vi "Sos_2024.vi"(0 "Temperature (K)":dbl=293.15 format="%.4g", 2 "Type of air":i32(listbox)=4, 5 "CO2 content (ppm)":dbl=500.0, 8 "Pressure (Pa)":dbl=101325.0 format="%.1f", 10 "xw molar fraction water vapor":dbl format="%.7g", 15 "Frequency (Hz)":dbl) -> (3 "virial correction Kv (ppm)":dbl=506.9979263453592, 6 "heat capacity correction Kc (ppm)":dbl=-1069.8067159622403 format="%.1f", 7 "relaxation correction Kr (ppm)":dbl=258.42726337360375 format="%#.0f", 12 "simple speed of sound":dbl=344.29226419685074 format="%.4f", 13 "heat & virial & relax corrected speed of sound humid air":dbl=344.2397436562656 format="%.4f", 14 "heat capacity corrected speed of sound [m/s]":dbl=344.10805182751363 format="%.4f", 17 "heat capacity & virial corrected speed of sound":dbl=344.19527180818477 format="%.4f")   [LabVIEW 2016]
panel:
  # "m/s"
  # "m/s"
  # "m/s"
  # "m/s"
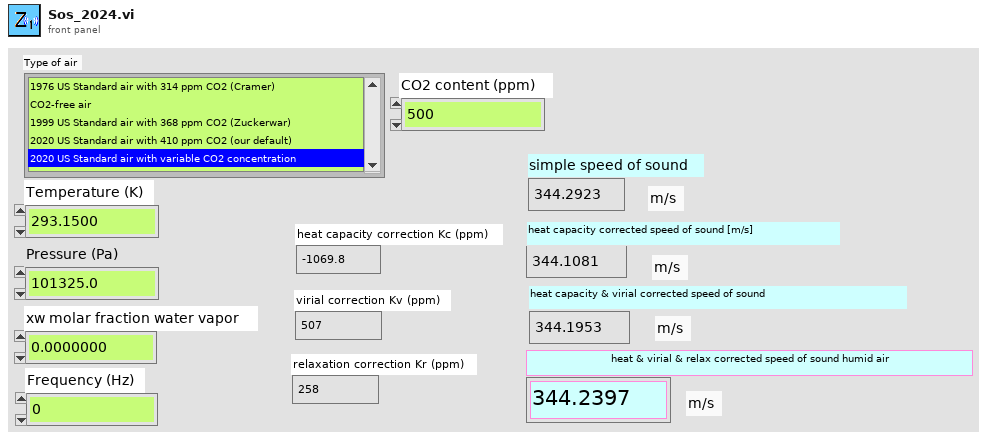
[diagram p1: front panel]
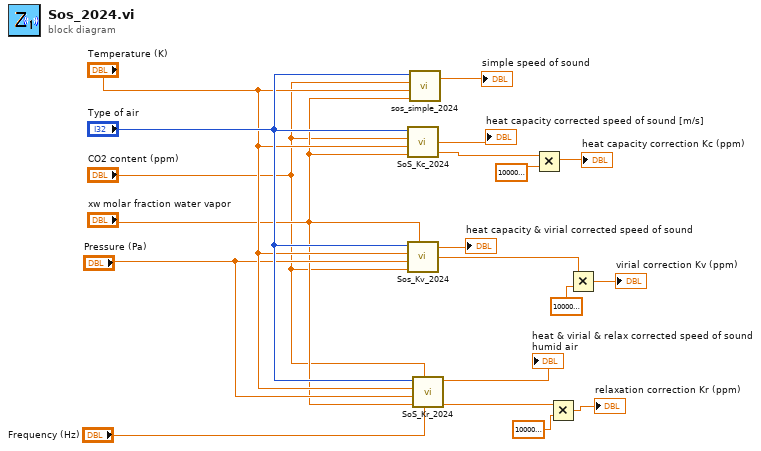
[diagram p0: block diagram]
diagram:
  n1 = call "SoS_Kc_2024.vi"("xw H2O molar fraction"="xw molar fraction water vapor", "Temperature [K]"="Temperature (K)", "CO2 content (ppm)"="CO2 content (ppm)", "Type of air"="Type of air") -> ("Kc"=w10:dbl, "Sos gamma0RT/M check [m/s]"=→"heat capacity corrected speed of sound [m/s]":dbl)  [unwired: 1 out]
  n2 = call "Sos_Kv_2024.vi"("Type of air"="Type of air", "Temperature (K)"="Temperature (K)", "Pressure (Pa)"="Pressure (Pa)", "CO2 content (ppm)"="CO2 content (ppm)", "xw molar fraction water vapor"="xw molar fraction water vapor") -> ("Sos Kv (m/s)"=→"heat capacity & virial corrected speed of sound":dbl, "Kv"=w12:dbl)  [unwired: 1 in]
  n3 = call "sos_simple_2024.vi"("xw H2O molar fraction"="xw molar fraction water vapor", "Temperature [K]"="Temperature (K)", "CO2 content (ppm)"="CO2 content (ppm)", "Type of air"="Type of air") -> ("Simple speed of sound  correct [m/s]"=→"simple speed of sound":dbl)  [unwired: 1 out]
  n4 = call "SoS_Kr_2024.vi"("Frequency (Hz)"="Frequency (Hz)", "CO2 content (ppm)"="CO2 content (ppm)", "xw molar fraction water vapor"="xw molar fraction water vapor", "Pressure (Pa)"="Pressure (Pa)", "Temperature (K)"="Temperature (K)", "Type of air"="Type of air") -> ("Kr"=w5:dbl, "Heat capacity, virial and relax corr speed of sound [m/s]"=→"heat & virial & relax corrected speed of sound humid air":dbl)  [unwired: 1 in, 1 out]
  n5 = Multiply(x=w10, y=1000000.0) -> (x*y=→"heat capacity correction Kc (ppm)":dbl)
  n6 = Multiply(x=w5, y=1000000.0) -> (x*y=→"relaxation correction Kr (ppm)":dbl)
  n7 = Multiply(x=w12, y=1000000.0) -> (x*y=→"virial correction Kv (ppm)":dbl)
